vi "Update.vi"(11 "Simple Actor in":refnum<class "Simple Actor.lvclass">) -> (3 "Simple Actor out":refnum<class "Simple Actor.lvclass">)   [LabVIEW 2017, in "Simple Actor.lvlib" / "Simple Actor.lvclass"]
uses:
  Simple Actor.lvclass
  Simple Actor.lvclass/Simple Actor.ctl
  <vilib>/ptbypt/NI_PtbyPt.lvlib
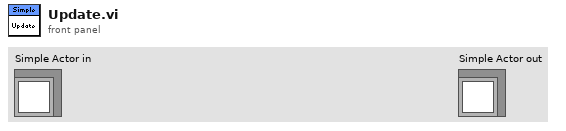
[diagram p1: front panel]
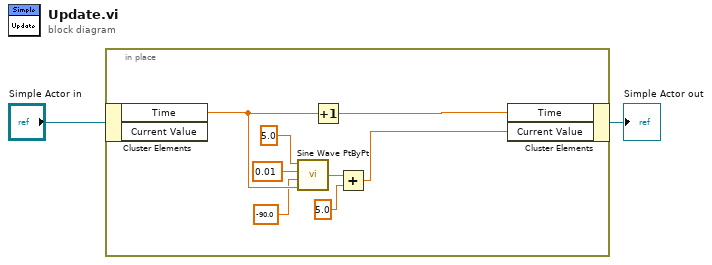
[diagram p0: block diagram]
diagram:
  n1 = in-place {
    n2 = in-place-cluster #1("Simple Actor in") -> ("Time"=w7:dbl)  [unwired: 1 out]
    n3 = call <vilib>:"Sine Wave PtByPt.vi"("time"=w7, "phase"=-90.0, "frequency"=0.01, "amplitude"=5.0) -> ("sine wave"=w8:dbl)
    n4 = Increment(x=w7) -> (x+1=w6:dbl)
    n5 = Add(x=w8, y=5.0) -> (x+y=w3:dbl)
    n6 = in-place-cluster #1("Time"=w6, "Current Value"=w3) -> (→"Simple Actor out":refnum<class "Simple Actor.lvclass">)
  }
